vi "GetLibraryItems.vi"(8 "error in (no error)":errorcluster, 11 "LVLibrary":refnum<vi>) -> (0 "error out":errorcluster, 2 "Names":string[](array[string]), 3 "Item Paths":path[](array[path]))   [LabVIEW 2020, in "ConstantErrorsMaker.lvlib"]
uses:
  ConstantErrorsMaker.lvlib
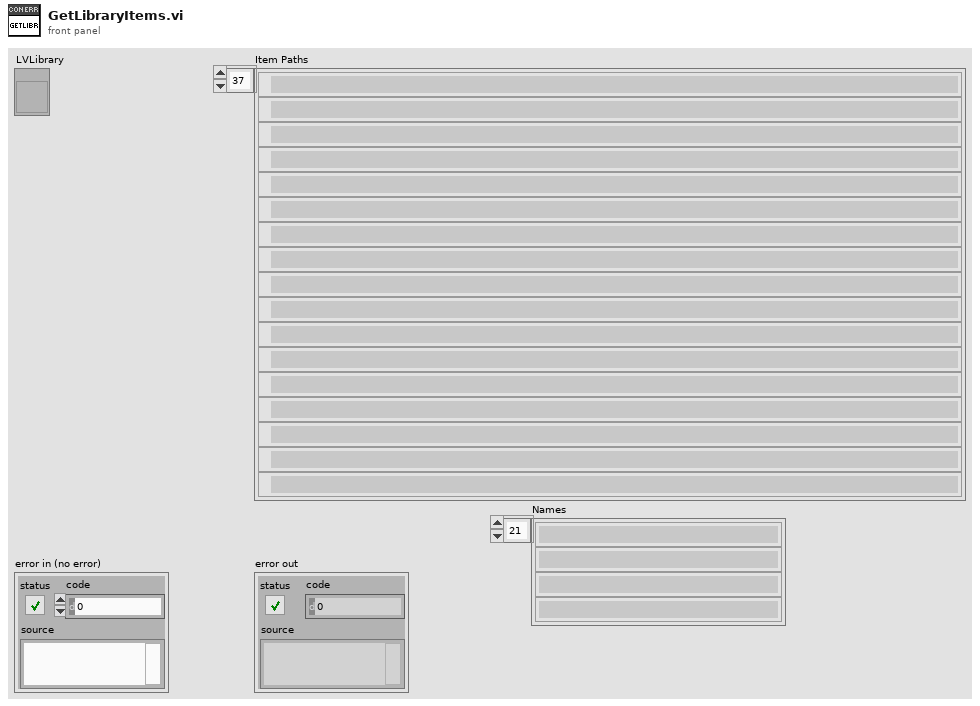
[diagram p1: front panel]
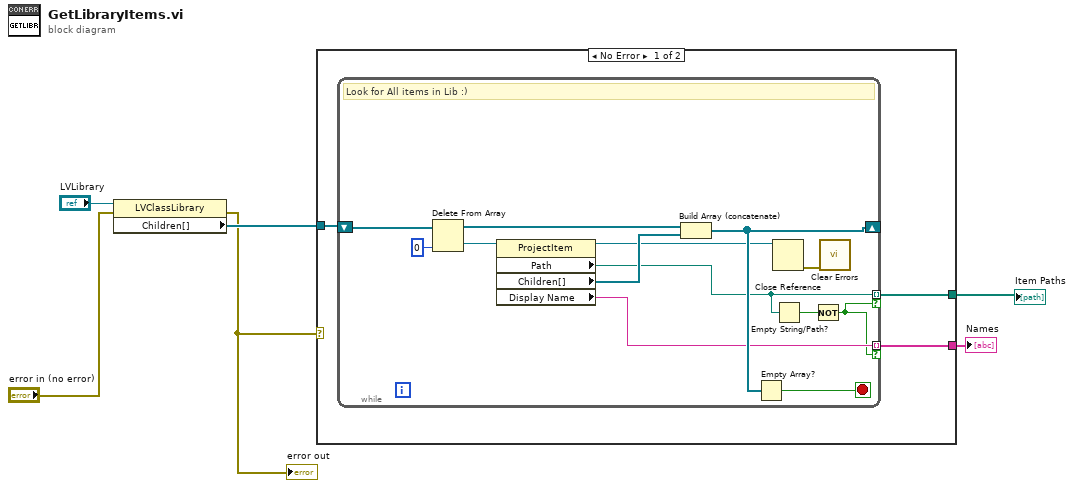
[diagram p0: block diagram]
diagram:
  n1 = property class="LVClassLibrary"(reference="LVLibrary", error in="error in (no error)") -> (error out=w4:errorcluster, "Children[]"=w6:refnum<vi>[])  [unwired: 1 out]
  "error out" <- w4
  n2 = case shown="No Error" w4 {
    tunnel: w6 -> [w9 _]
    tunnel: [w8 _] -> w5
    tunnel: [w7 _] -> w2
    frame No Error {
      n3 = while {
        shift-right: [w18] -> _
        shift-left: w9 -> [w22]
        tunnel: [w15] -> w8 mode=indexing if=w11
        tunnel: [w12] -> w7 mode=indexing if=w11
        stop <- w17 stop-if-true
        # "Look for All items in Lib :)"
        n4 = Delete From Array(array=w22, index=0) -> (deleted portion=w20:refnum<vi>, array with subset deleted=w10:refnum<vi>[])  [unwired: 1 in]
        n5 = property class="ProjectItem"(reference=w20) -> (reference out=w16:refnum<vi>, "Path"=w15:path, "Children[]"=w19:refnum<vi>[], "Display Name"=w12:string)  [unwired: 1 in, 1 out]
        n6 = Build Array (concatenate)(w10, w19) -> (w18:refnum<vi>[])
        n7 = Empty Array?(array=w18) -> (empty?=w17:bool)
        n8 = Close Reference(reference=w16) -> (error out=w13:errorcluster)  [unwired: 1 in]
        n9 = Empty String/Path?(string/path=w15) -> (empty?=w14:bool)
        n10 = Not(x=w14) -> (.not. x?=w11:bool)
        n11 = call <vilib>:"Clear Errors.vi"("error in (no error)"=w13) -> ()  [unwired: 5 in, 2 out]
      }
    }
    frame Error {
    }
  }
  "Item Paths" <- w5
  "Names" <- w2
